vi "Terminals Msg Input Relation.vi"(10 "Terminals (Msg Input)":T1) -> (2 "Terminals (Msg Input) Relation":T1)   [LabVIEW 2020, in "_Rescript.lvlib" / "Msg.lvlib" / "Msg.lvclass"]
uses:
  Msg.lvclass
  Terminals.ctl
  _Rescript.lvlib
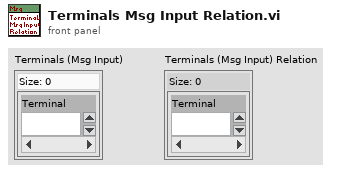
[diagram p1: front panel]
types:
  T1 = typedef "_Rescript.lvlib/Terminals.ctl" = set{i32}
  T2 = typedef "_Rescript.lvlib/Msg.lvlib/Msg.lvclass/Terminal Relation.ctl" = map{i32, i32}
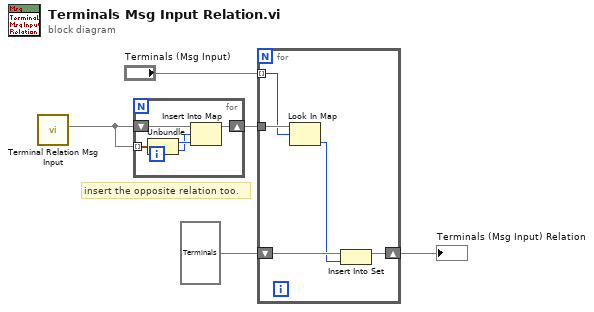
[diagram p0: block diagram]
diagram:
  # "insert the opposite relation too."
  n1 = call "Terminal Relation Msg Input.vi"() -> ("Terminal Relation (Msg Input)"=w1:T2)  [unwired: 11 in]
  n2 = for {
    shift-right: [w9] -> w2
    shift-left: w1 -> [w10]
    tunnel: w1 -> [w8] mode=indexing
    n3 = Unbundle(w8) -> ("Terminal"=w7:i32, "Terminal"=w6:i32)
    n4 = Insert Into Map(map in=w10, key=w6, value=w7) -> (map out=w9:T2)  [unwired: 2 out]
  }
  n5 = for {
    tunnel: "Terminals (Msg Input)" -> [w14] mode=indexing
    tunnel: w2 -> [w15]
    shift-right: [w12] -> w4
    shift-left: T1 {} ("Terminals (Read Msg Input)") -> [w13]
    n6 = Look In Map(map=w15, key=w14) -> (value=w11:i32)  [unwired: 1 in, 1 out]
    n7 = Insert Into Set(10:w11, 11:w13) -> (3:w12:T1)  [unwired: 1 out]
  }
  "Terminals (Msg Input) Relation" <- w4
